vi "Update Dynamic Sensor Displays.vi"(7 "Sensor Data":T2[](array[typedef]) {"Value" scale=0.0..10.0}, 10 "Sensor List":T1[](array[typedef]), 11 "Control List List":refnum<vi>[][](array[refnum])) -> ()   [LabVIEW 2015]
uses:
  Transducer Calibration Display.ctl
  Sensor Enum.ctl
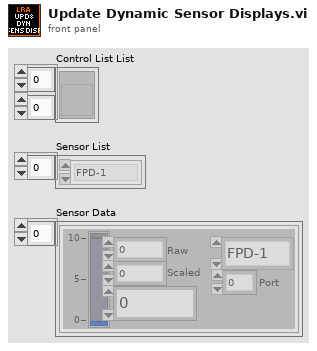
[diagram p1: front panel]
types:
  T1 = typedef "Sensor Enum.ctl" = enum16{"FPD-1", "FPD-2", "FPD-3", "OPD-1", "OPD-2", "OPD-3", "AP-1", "PC-1", "PC-2", "VBAT", "VCOMP", "ICOMP", "TC-1", "TC-COMP"}
  T2 = typedef "Transducer Calibration Display.ctl" = cluster{"Value":dbl, "Raw":dbl, "Scaled":dbl, "Sensor Name":T1, "Port":u32}
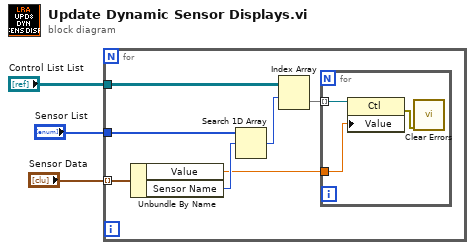
[diagram p0: block diagram]
diagram:
  n1 = for {
    tunnel: "Sensor List" -> [w9]
    tunnel: "Control List List" -> [w6]
    tunnel: "Sensor Data" -> [w10] mode=indexing
    n2 = Unbundle By Name(w10) -> ("Value"=w4:dbl, "Sensor Name"=w8:T1)
    n3 = Search 1D Array(1D array=w9, element=w8) -> (index of element=w7:i32)  [unwired: 1 in]
    n4 = Index Array(array=w6, index (row)=w7) -> (element=w5:refnum<vi>[])  [unwired: 1 in]
    n5 = for {
      tunnel: w5 -> [w13] mode=indexing
      tunnel: w4 -> [w12]
      n6 = property class="Ctl"(reference=w13, "Value"=w12) -> (error out=w11:errorcluster)  [unwired: 1 in, 1 out]
      n7 = call <vilib>:"Clear Errors.vi"("error in (no error)"=w11) -> ()  [unwired: 5 in, 2 out]
    }
  }
